vi "PathPlanner_PathFinder_GetWorkerStatus.vi"() -> (3 "PathFindingWorkerStatus":T1)   [LabVIEW 2019, in "PathPlanner24.lvlib"]
doc: "Get status of Path Finder worker"
uses:
  PathPlanner24.lvlib
  PathPlanner_PathFinder_Globals.vi
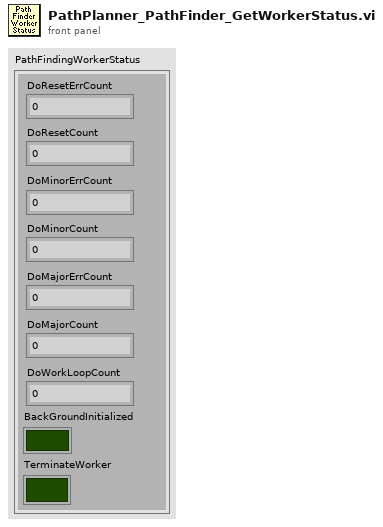
[diagram p1: front panel]
types:
  T1 = cluster{"DoResetErrCount":i64, "DoResetCount":i64, "DoMinorErrCount":i64, "DoMinorCount":i64, "DoMajorErrCount":i64, "DoMajorCount":i64, "DoWorkLoopCount":i64, "BackGroundInitialized":bool, "TerminateWorker":bool}
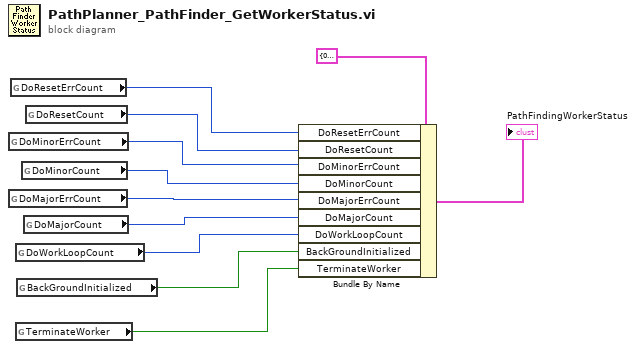
[diagram p0: block diagram]
diagram:
  n1 = global read "PathPlanner_PathFinder_Globals.vi" "DoMinorErrCount"() -> (w3:i64)
  n2 = global read "PathPlanner_PathFinder_Globals.vi" "DoMajorErrCount"() -> (w5:i64)
  n3 = global read "PathPlanner_PathFinder_Globals.vi" "DoResetErrCount"() -> (w1:i64)
  n4 = global read "PathPlanner_PathFinder_Globals.vi" "DoWorkLoopCount"() -> (w7:i64)
  n5 = global read "PathPlanner_PathFinder_Globals.vi" "TerminateWorker"() -> (w9:bool)
  n6 = global read "PathPlanner_PathFinder_Globals.vi" "BackGroundInitialized"() -> (w8:bool)
  n7 = global read "PathPlanner_PathFinder_Globals.vi" "DoMinorCount"() -> (w4:i64)
  n8 = global read "PathPlanner_PathFinder_Globals.vi" "DoMajorCount"() -> (w6:i64)
  n9 = global read "PathPlanner_PathFinder_Globals.vi" "DoResetCount"() -> (w2:i64)
  n10 = Bundle By Name(cluster=T1 {"DoResetErrCount"=0, "DoResetCount"=0, "DoMinorErrCount"=0, "DoMinorCount"=0, "DoMajorErrCount"=0, "DoMajorCount"=0, "DoWorkLoopCount"=0, "BackGroundInitialized"=FALSE, "TerminateWorker"=FALSE} ("PathFindingWorkerStatus"), "DoResetErrCount"=w1, "DoResetCount"=w2, "DoMinorErrCount"=w3, "DoMinorCount"=w4, "DoMajorErrCount"=w5, "DoMajorCount"=w6, "DoWorkLoopCount"=w7, "BackGroundInitialized"=w8, "TerminateWorker"=w9) -> (→"PathFindingWorkerStatus":T1)
